vi "Read System Queue.vi"(8 "error in (no error)":errorcluster, 11 "Receiver Command in":refnum<class "Receiver Command.lvclass">) -> (0 "error out":errorcluster, 2 "Actor Framework:Message Enqueuer":refnum<class "Message Enqueuer.lvclass">, 3 "Receiver Command out":refnum<class "Receiver Command.lvclass">)   [LabVIEW 2013, in "Receiver.lvlib" / "Receiver Commands using Actor.lvlib" / "Receiver Command.lvclass"]
uses:
  Receiver Command.lvclass
  <vilib>/ActorFramework/Message Enqueuer/Message Enqueuer.lvclass
  Receiver Command.lvclass/Receiver Command.ctl
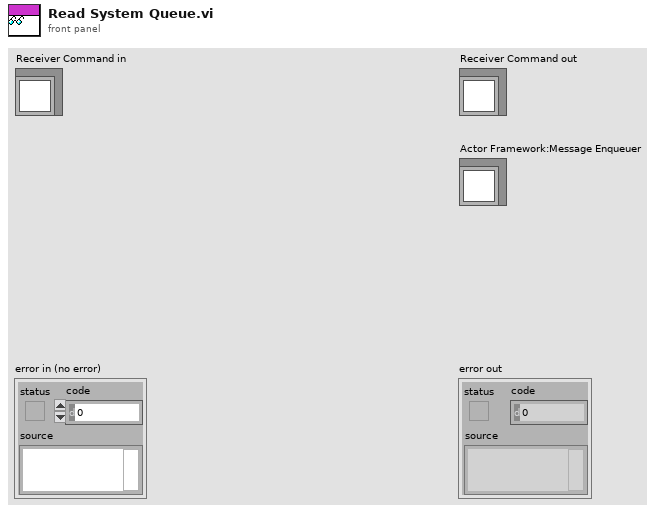
[diagram p1: front panel]
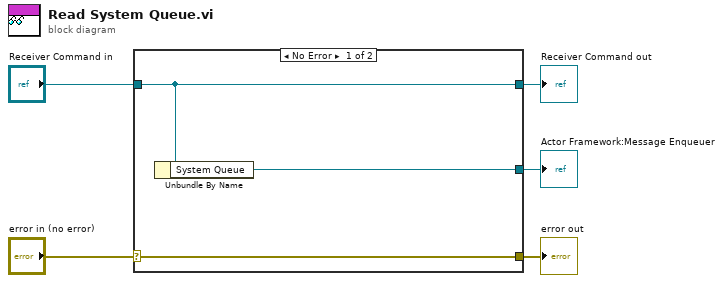
[diagram p0: block diagram]
diagram:
  n1 = case shown="No Error" "error in (no error)" {
    selector: "error in (no error)" -> [w8 w9]
    tunnel: [w8 w9] -> w4
    tunnel: [w7 w10] -> w2
    tunnel: "Receiver Command in" -> [w7 w10]
    tunnel: [w6 _] -> w1
    frame No Error {
      n2 = Unbundle By Name(w7) -> ("System Queue"=w6:refnum<class "Message Enqueuer.lvclass">)
    }
    frame Error {
    }
  }
  "error out" <- w4
  "Receiver Command out" <- w2
  "Actor Framework:Message Enqueuer" <- w1
